vi "Get Scanimage Frame.vi"(8 "error in":errorcluster, 11 "Image":T1) -> (0 "error out":errorcluster, 3 "Image":T1(plugin-control))   [LabVIEW 2012, in "Sciscan Scope Daemon.lvlib"]
uses:
  <vilib>/vision/Image Controls.llb/IMAQ Image.ctl
  Sciscan Scope Daemon.lvlib
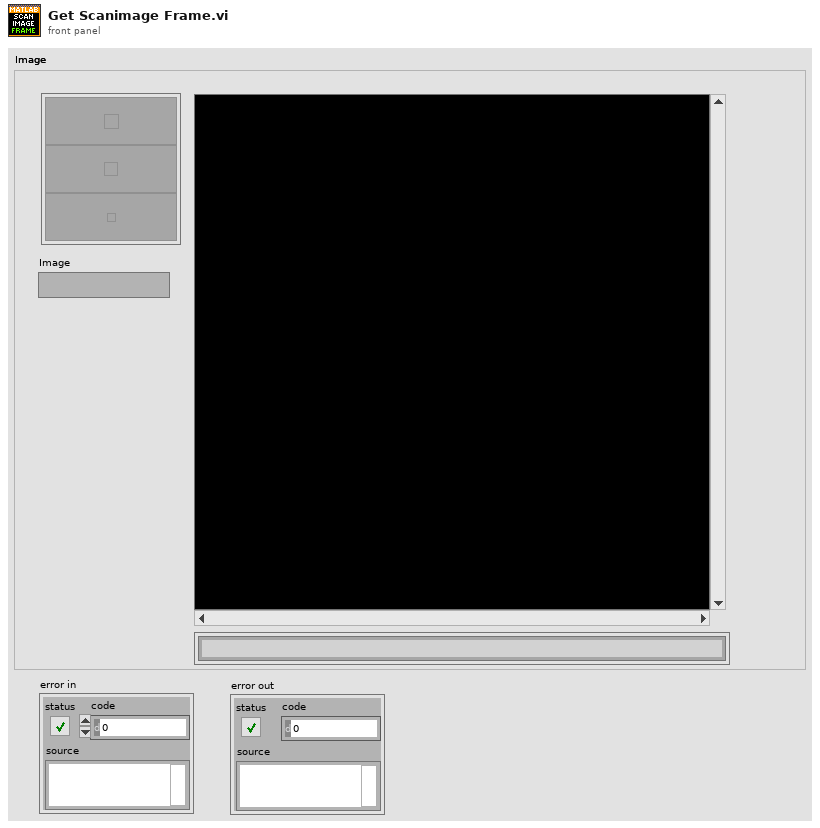
[diagram p1: front panel]
types:
  T1 = typedef "IMAQ Image.ctl" = refnum<image>
  T2 = cluster{u16, u16, "Plane 4 (alpha)":u16, "Plane 4 (alpha)":u16}
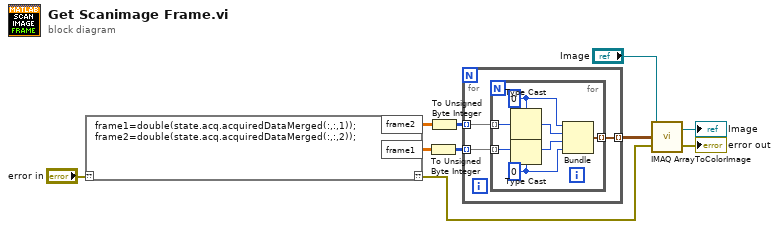
[diagram p0: block diagram]
diagram:
  n1 = script code="frame1=double(state.acq.acquiredDataMerged(:,:,1)); \nframe2=double(state.acq.acquiredDataMerged(:,:,2));"("??"="error in") -> ("??"=w3:errorcluster, "frame2"=w8:dbl[][], "frame1"=w9:dbl[][])
  n2 = To Unsigned Byte Integer(number=w9) -> (unsigned 8bit integer=w6:u8[][])
  n3 = To Unsigned Byte Integer(number=w8) -> (unsigned 8bit integer=w7:u8[][])
  n4 = for {
    tunnel: w6 -> [w13] mode=indexing
    tunnel: [w12] -> w2 mode=indexing
    tunnel: w7 -> [w11] mode=indexing
    n5 = for {
      tunnel: w13 -> [w18] mode=indexing
      tunnel: [w20] -> w12 mode=indexing
      tunnel: w11 -> [w19] mode=indexing
      w15 = u16 0
      w14 = u16 0 ("Plane 4 (alpha)")
      n6 = Type Cast(type=w15, x=w19) -> (*(type *) &x=w16:u16)
      n7 = Type Cast(type=w14, x=w18) -> (*(type *) &x=w17:u16)
      n8 = Bundle(w15, w16, "Plane 4 (alpha)"=w17, "Plane 4 (alpha)"=w14) -> (w20:T2)  [unwired: 1 in]
    }
  }
  n9 = call "IMAQ ArrayToColorImage"("Image"="Image", "Image Pixels (U64)"=w2, "error in (no error)"=w3) -> ("Image Out"=→"Image":T1, "error out"=→"error out":errorcluster)  [unwired: 2 in]
